vi "Flat Img To 24 Bit.vi"(1 "image data":T1) -> (0 "24-bit pixmap":u32[][](array[numeric]))   [LabVIEW 2020]
uses:
  <vilib>/picture/picture.llb/imagedata.ctl
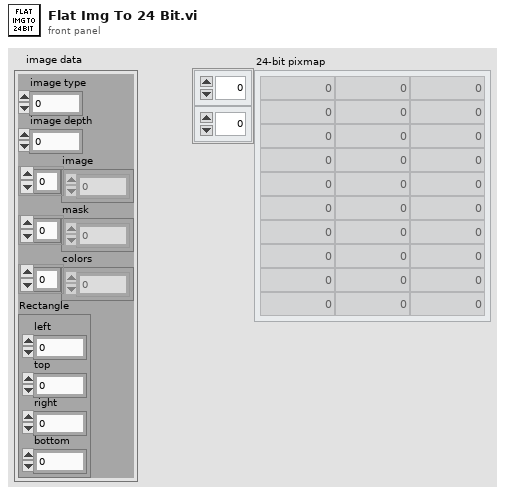
[diagram p1: front panel]
types:
  T1 = typedef "imagedata.ctl" = cluster{"image type":i32, "image depth":i32, "image":u8[], "mask":u8[], "colors":u32[], "Rectangle":cluster{"left":i16, "top":i16, "right":i16, "bottom":i16}}
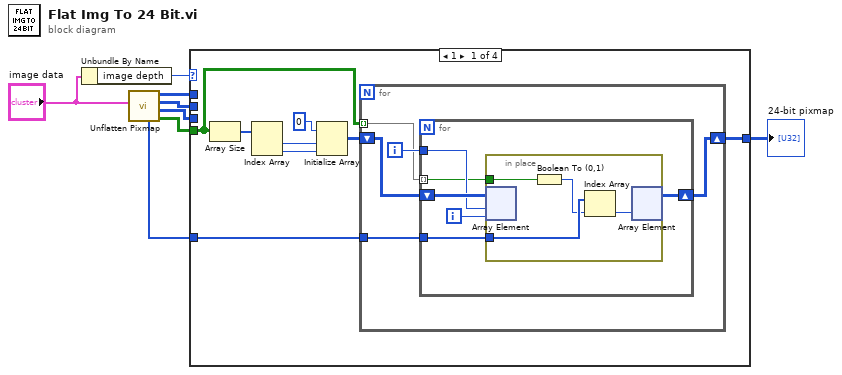
[diagram p0: block diagram]
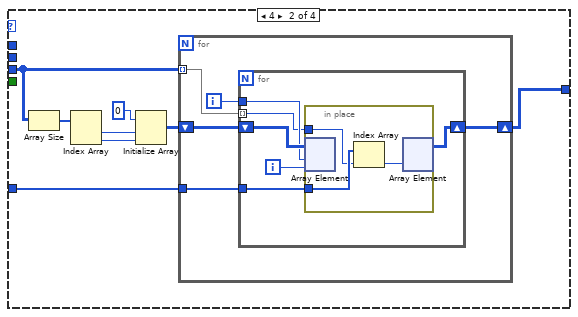
[diagram p2: hidden frame]
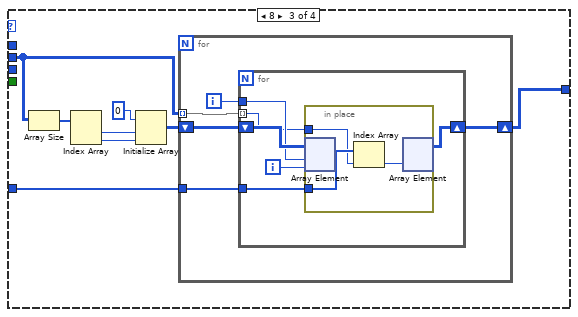
[diagram p3: hidden frame]
diagram:
  n1 = Unbundle By Name("image data") -> ("image depth"=w7:i32)
  n2 = call <vilib>:"Unflatten Pixmap.vi"("image data"="image data") -> ("1-bit pixmap"=w6:bool[][], "4-bit pixmap"=w4:u8[][], "8-bit pixmap"=w3:u8[][], "24-bit pixmap"=w2:u32[][], "colors"=w5:u32[])  [unwired: 4 in, 2 out]
  n3 = case shown="1" w7 {
    tunnel: w6 -> [w9 _ _ _]
    tunnel: w5 -> [w16 w39 w61 _]
    tunnel: [w10 w33 w55 w76] -> w1
    tunnel: w4 -> [_ w32 _ _]
    tunnel: w3 -> [_ _ w54 _]
    tunnel: w2 -> [_ _ _ w76]
    frame 1 {
      n4 = Array Size(array=w9) -> (size(s)=w14:i32[])
      n5 = Index Array(array=w14) -> (element #1=w13:i32, element #2=w12:i32)  [unwired: 2 in]
      n6 = Initialize Array(u32 0, w13, w12) -> (w11:u32[][])
      n7 = for {
        tunnel: w16 -> [w21]
        shift-right: [w20] -> w10
        shift-left: w11 -> [w19]
        tunnel: w9 -> [w17] mode=indexing
        i -> [w18]
        n8 = for {
          tunnel: w21 -> [w23]
          shift-right: [w26] -> w20
          shift-left: w19 -> [w27]
          tunnel: w18 -> [w25]
          tunnel: w17 -> [w22] mode=indexing
          i -> [w24]
          n9 = in-place {
            in-place-border: w23 -> [w31]
            in-place-border: w22 -> [w29]
            n10 = in-place-array #1(w27, w25, w24) -> ()  [unwired: 1 out]
            n11 = Boolean To (0,1)(Boolean=w29) -> (0, 1=w28:i16)
            n12 = Index Array(array=w31, index=w28) -> (element=w30:u32)
            n13 = in-place-array #1(w30) -> (w26:u32[][])  [unwired: 2 out]
          }
        }
      }
    }
    frame 4 {
      n14 = Array Size(array=w32) -> (size(s)=w37:i32[])
      n15 = Index Array(array=w37) -> (element #1=w36:i32, element #2=w35:i32)  [unwired: 2 in]
      n16 = Initialize Array(u32 0, w36, w35) -> (w34:u32[][])
      n17 = for {
        tunnel: w32 -> [w44] mode=indexing
        tunnel: w39 -> [w43]
        shift-right: [w42] -> w33
        shift-left: w34 -> [w41]
        i -> [w40]
        n18 = for {
          tunnel: w44 -> [w45] mode=indexing
          tunnel: w43 -> [w46]
          shift-right: [w49] -> w42
          shift-left: w41 -> [w50]
          tunnel: w40 -> [w48]
          i -> [w47]
          n19 = in-place {
            in-place-border: w46 -> [w53]
            in-place-border: w45 -> [w52]
            n20 = in-place-array #2(w50, w48, w47) -> ()  [unwired: 1 out]
            n21 = Index Array(array=w53, index=w52) -> (element=w51:u32)
            n22 = in-place-array #2(w51) -> (w49:u32[][])  [unwired: 2 out]
          }
        }
      }
    }
    frame 8 {
      n23 = Array Size(array=w54) -> (size(s)=w59:i32[])
      n24 = Index Array(array=w59) -> (element #1=w58:i32, element #2=w57:i32)  [unwired: 2 in]
      n25 = Initialize Array(u32 0, w58, w57) -> (w56:u32[][])
      n26 = for {
        tunnel: w54 -> [w66] mode=indexing
        tunnel: w61 -> [w65]
        shift-right: [w64] -> w55
        shift-left: w56 -> [w63]
        i -> [w62]
        n27 = for {
          tunnel: w66 -> [w67] mode=indexing
          tunnel: w65 -> [w68]
          shift-right: [w71] -> w64
          shift-left: w63 -> [w72]
          tunnel: w62 -> [w70]
          i -> [w69]
          n28 = in-place {
            in-place-border: w68 -> [w75]
            in-place-border: w67 -> [w74]
            n29 = in-place-array #3(w72, w70, w69) -> ()  [unwired: 1 out]
            n30 = Index Array(array=w75, index=w74) -> (element=w73:u32)
            n31 = in-place-array #3(w73) -> (w71:u32[][])  [unwired: 2 out]
          }
        }
      }
    }
    frame 24, Default {
    }
  }
  "24-bit pixmap" <- w1
